vi "Status Updated.vi"(8 "error in":errorcluster, 10 "Status":string, 11 "Module ID":i32=-1) -> (0 "error out":errorcluster)   [LabVIEW 2018, in "ModuleInterface.lvlib"]
doc: "Send the Status Updated event to any VI registered to listen to events from the owning module.\n_____\nBased on DQMH Project Template 7.0.1.1316."
uses:
  ModuleInterface.lvlib
  Status Updated Argument--cluster.ctl
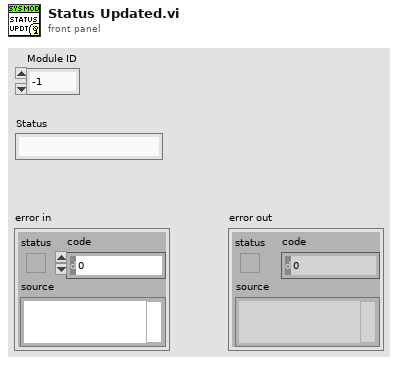
[diagram p1: front panel]
types:
  T1 = typedef "ModuleInterface.lvlib/Status Updated Argument--cluster.ctl" = cluster{"Status":string, "Module ID":i32}
  T2 = typedef "ModuleInterface.lvlib/Broadcast Events--cluster.ctl" = cluster{"Module Did Init":refnum<user-event>, "Status Updated":refnum<user-event>, "Error Reported":refnum<user-event>, "Module Did Stop":refnum<user-event>, "Update Module Execution Status":refnum<user-event>, "Function Selected":refnum<user-event>, "Window Size Changed":refnum<user-event>}
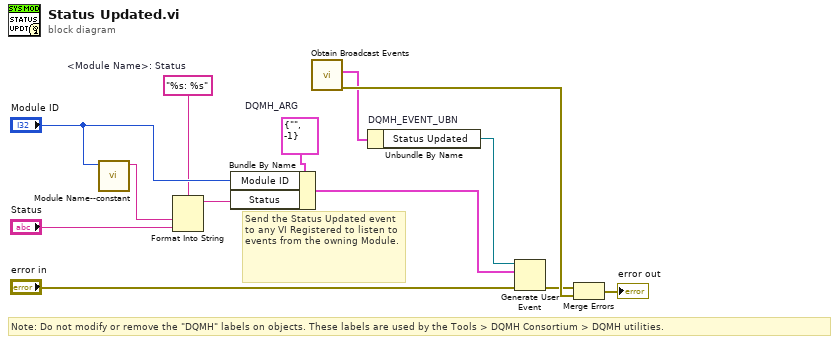
[diagram p0: block diagram]
diagram:
  w4 = "%s: %s"  # <Module Name>: Status
  w7 = T1 {"Status"="", "Module ID"=-1}  # DQMH_ARG
  # "Note: Do not modify or remove the \"DQMH\" labels on objects. These labels are used by the Tools > DQMH Consortium > DQMH utilities."
  # "Send the Status Updated event to any VI Registered to listen to events from the owning Module."
  n1 = call "Module Name--constant.vi"("Module ID"="Module ID") -> ("Module Name"=w3:string)  [unwired: 10 in]
  n2 = Format Into String(format string=w4, w3, "Status") -> (resulting string=w1:string)  [unwired: 2 in, 1 out]
  n3 = Bundle By Name(cluster=w7, "Module ID"="Module ID", "Status"=w1) -> (w6:T1)
  n4 = call "Obtain Broadcast Events.vi"() -> ("error out"=w11:errorcluster, "ModuleInterface Broadcast Events"=w9:T2)  [unwired: 10 in]
  n5 = Unbundle By Name "DQMH_EVENT_UBN"(w9) -> ("Status Updated"=w8:refnum<user-event>)
  n6 = Generate User Event(user event=w8, event data cluster=w6, error in="error in") -> (error out=w10:errorcluster)  [unwired: 1 in, 1 out]
  n7 = Merge Errors(w10, w11) -> (→"error out":errorcluster)
